vi "Monitor voltages.vi"() -> ()   [LabVIEW 2020]
uses:
  <vilib>/Utility/error.llb/DialogType.ctl
  <vilib>/DAQmx/read.llb/DAQmx Read (Analog 1D Wfm NChan NSamp).vi
  <vilib>/DAQmx/create/channels.llb/DAQmx Create Channel (AI-Voltage-Basic).vi
  <vilib>/DAQmx/configure/timing.llb/DAQmx Timing (Sample Clock).vi
  <vilib>/DAQmx/miscellaneous.llb/DAQmx Fill In Error Info.vi
  <vilib>/Utility/file.llb/Write Delimited Spreadsheet (DBL).vi
  <resource>/objmgr/daqmx.rc
  <vilib>/Analysis/NI_AALBase.lvlib
panel:
  out "Waveform Chart":cluster{"[0]":dbl, "[1]":dbl, "[2]":dbl}(graph)
  out "STD":dbl[](array[numeric])=[0.0007136534746484955, 0.0006582648996476653, 0.0006977354612249226]
  out "Mean voltage":dbl[](array[numeric])=[-1.226623991867514, -1.2306075649591512, -1.3978613305300918]
  in  "Log data":bool
  in  "Logging period (s)":dbl=1.0 caption="Time Target (s)"
  out "Waveform Graph":waveform(dbl)[](graph)=[{"t0"=timestamp(3798561010.450787 s since 1904-01-01), "dt"=0.001, "Y"=[-1.2267769584961297, -1.2264549234868314, -1.2259718709735348, -1.2267769584961297, -1.2254888184610193, -1.227904081031412, -1.2256498359651042, -1.2254888184610193, -1.2270989935057757, -1.227904081031412, -1.2264549234868314, -1.226615940991437, -1.226615940991437, -1.2275820460208966, -1.226615940991437, -1.2250057659492843, -1.2280650985368, -1.226615940991437, -1.2258108534692762, -1.2269379760009091, -1.2274210285157692, -1.2269379760009091, -1.2261328884778802, -1.2264549234868314, -1.2270989935057757, -1.2264549234868314, -1.2274210285157692, -1.2261328884778802, -1.2269379760009091, -1.2261328884778802, -1.2264549234868314, -1.2280650985368, -1.2264549234868314, -1.2267769584961297, -1.2270989935057757, -1.2269379760009091, -1.2267769584961297, -1.2270989935057757, -1.2259718709735348, -1.2269379760009091, -1.227260011010729, -1.2259718709735348, -1.2262939059823121, -1.2270989935057757, -1.2269379760009091, -1.226615940991437, -1.2259718709735348, -1.226615940991437, -1.2267769584961297, -1.2264549234868314, -1.2250057659492843, -1.2254888184610193, -1.2270989935057757, -1.2262939059823121, -1.225327800957021, -1.2277430635261108, -1.227260011010729, -1.2258108534692762, -1.2254888184610193, -1.2261328884778802, -1.2262939059823121, -1.2270989935057757, -1.2261328884778802, -1.227260011010729, -1.2254888184610193, -1.2258108534692762, -1.2277430635261108, -1.2280650985368, -1.2270989935057757, -1.2262939059823121, -1.2264549234868314, -1.226615940991437, -1.2264549234868314, -1.2269379760009091, -1.2269379760009091, -1.227904081031412, -1.2275820460208966, -1.2264549234868314, -1.2267769584961297, -1.2270989935057757, -1.2267769584961297, -1.2259718709735348, -1.2264549234868314, -1.2277430635261108, -1.2251667834531093, -1.2254888184610193, -1.2264549234868314, -1.2267769584961297, -1.2270989935057757, -1.2250057659492843, -1.2274210285157692, -1.226615940991437, -1.2264549234868314, -1.226615940991437, -1.2262939059823121, -1.2269379760009091, -1.226615940991437, -1.226615940991437, -1.2274210285157692, -1.2267769584961297], "attributes"=variant("NI_ChannelName"=variant(string "Dev1/ai0"), "NI_UnitDescription"=variant(string "Volts"))}, {"t0"=timestamp(3798561010.450798 s since 1904-01-01), "dt"=0.001, "Y"=[-1.2311244311557337, -1.2311244311557337, -1.230802396141731, -1.2299973086082525, -1.2312854486628662, -1.230802396141731, -1.2312854486628662, -1.2316074836773934, -1.230319343621382, -1.2306413786348607, -1.230802396141731, -1.2309634136486887, -1.2301583261147735, -1.2304803611280777, -1.2314464661700861, -1.230802396141731, -1.229675273595472, -1.2312854486628662, -1.230802396141731, -1.2298362911018186, -1.2304803611280777, -1.2306413786348607, -1.2301583261147735, -1.230319343621382, -1.2309634136486887, -1.230319343621382, -1.2298362911018186, -1.2306413786348607, -1.2309634136486887, -1.2295142560892127, -1.2298362911018186, -1.2309634136486887, -1.2306413786348607, -1.2301583261147735, -1.231768501184788, -1.230319343621382, -1.2306413786348607, -1.2299973086082525, -1.2298362911018186, -1.230319343621382, -1.2295142560892127, -1.2319295186922703, -1.2316074836773934, -1.2309634136486887, -1.2304803611280777, -1.2312854486628662, -1.230802396141731, -1.2293532385830404, -1.2304803611280777, -1.2322515537074974, -1.2306413786348607, -1.230802396141731, -1.2309634136486887, -1.2311244311557337, -1.2306413786348607, -1.2295142560892127, -1.2304803611280777, -1.2309634136486887, -1.2299973086082525, -1.2304803611280777, -1.2304803611280777, -1.230802396141731, -1.230802396141731, -1.2309634136486887, -1.2309634136486887, -1.2298362911018186, -1.2301583261147735, -1.2306413786348607, -1.2299973086082525, -1.230319343621382, -1.230802396141731, -1.2309634136486887, -1.2299973086082525, -1.2301583261147735, -1.228870186065047, -1.231768501184788, -1.2306413786348607, -1.230319343621382, -1.2304803611280777, -1.2290312035709576, -1.2306413786348607, -1.2312854486628662, -1.2295142560892127, -1.2309634136486887, -1.2316074836773934, -1.230802396141731, -1.2298362911018186, -1.230319343621382, -1.23209053619984, -1.2312854486628662, -1.2295142560892127, -1.2306413786348607, -1.231768501184788, -1.230802396141731, -1.230802396141731, -1.2306413786348607, -1.2299973086082525, -1.2298362911018186, -1.2312854486628662, -1.2312854486628662], "attributes"=variant("NI_ChannelName"=variant(string "Dev1/ai1"), "NI_UnitDescription"=variant(string "Volts"))}, {"t0"=timestamp(3798561010.450809 s since 1904-01-01), "dt"=0.001, "Y"=[-1.3980996365889728, -1.398743707022256, -1.3976165837651384, -1.3974555661574082, -1.3982606541971323, -1.3977776013729755, -1.3997098126754064, -1.3982606541971323, -1.3977776013729755, -1.3979386189809204, -1.3980996365889728, -1.3980996365889728, -1.398582689413774, -1.3977776013729755, -1.3980996365889728, -1.3997098126754064, -1.3980996365889728, -1.3971335309422703, -1.3980996365889728, -1.3980996365889728, -1.3979386189809204, -1.396972513334862, -1.396972513334862, -1.3990657422395425, -1.3984216718053992, -1.395845390086009, -1.3963284429063025, -1.398582689413774, -1.3968114957275615, -1.3976165837651384, -1.3980996365889728, -1.396972513334862, -1.3976165837651384, -1.3979386189809204, -1.396972513334862, -1.3979386189809204, -1.3980996365889728, -1.3977776013729755, -1.3980996365889728, -1.3971335309422703, -1.398743707022256, -1.3980996365889728, -1.3982606541971323, -1.3977776013729755, -1.3982606541971323, -1.3972945485497856, -1.3977776013729755, -1.3980996365889728, -1.3974555661574082, -1.3972945485497856, -1.3990657422395425, -1.398582689413774, -1.3971335309422703, -1.3982606541971323, -1.3997098126754064, -1.3972945485497856, -1.396650478120368, -1.3977776013729755, -1.398743707022256, -1.3984216718053992, -1.3979386189809204, -1.3979386189809204, -1.3982606541971323, -1.3979386189809204, -1.398582689413774, -1.3989047246308455, -1.3971335309422703, -1.396972513334862, -1.3974555661574082, -1.3972945485497856, -1.3979386189809204, -1.398582689413774, -1.3976165837651384, -1.3972945485497856, -1.3971335309422703, -1.3979386189809204, -1.3974555661574082, -1.396972513334862, -1.3984216718053992, -1.3976165837651384, -1.3964894605132818, -1.3982606541971323, -1.398582689413774, -1.3977776013729755, -1.3971335309422703, -1.3974555661574082, -1.3974555661574082, -1.3976165837651384, -1.3977776013729755, -1.3989047246308455, -1.3976165837651384, -1.396972513334862, -1.3982606541971323, -1.3984216718053992, -1.3979386189809204, -1.3972945485497856, -1.3976165837651384, -1.3972945485497856, -1.3977776013729755, -1.398743707022256], "attributes"=variant("NI_ChannelName"=variant(string "Dev1/ai2"), "NI_UnitDescription"=variant(string "Volts"))}]
  in  "Stop":bool
  in  "Number of Samples":i32=100
  in  "Save File Path":path=path "G:/Shared drives/PHYS - Walsworth Group/Experiment folders/Dark Matter/Confocal/Data/Nanostage monitoring/test.lvm"
  in  "Sample Rate":dbl=1000.0
  in  "Sample Clock Source":tag="OnboardClock"
  in  "Terminal Configuration":i32(ring)=-1 items=["default"=-1, "RSE"=10083, "NRSE"=10078, "Differential"=10106, "Pseudodifferential"=12529]
  in  "Max Voltage":dbl=10.0
  in  "Min Voltage":dbl=-10.0
  in  "Physical Channel":tag="Dev1/ai0:2"
  out "Actual Sample Rate":dbl=1000.0 format="%0.2f"
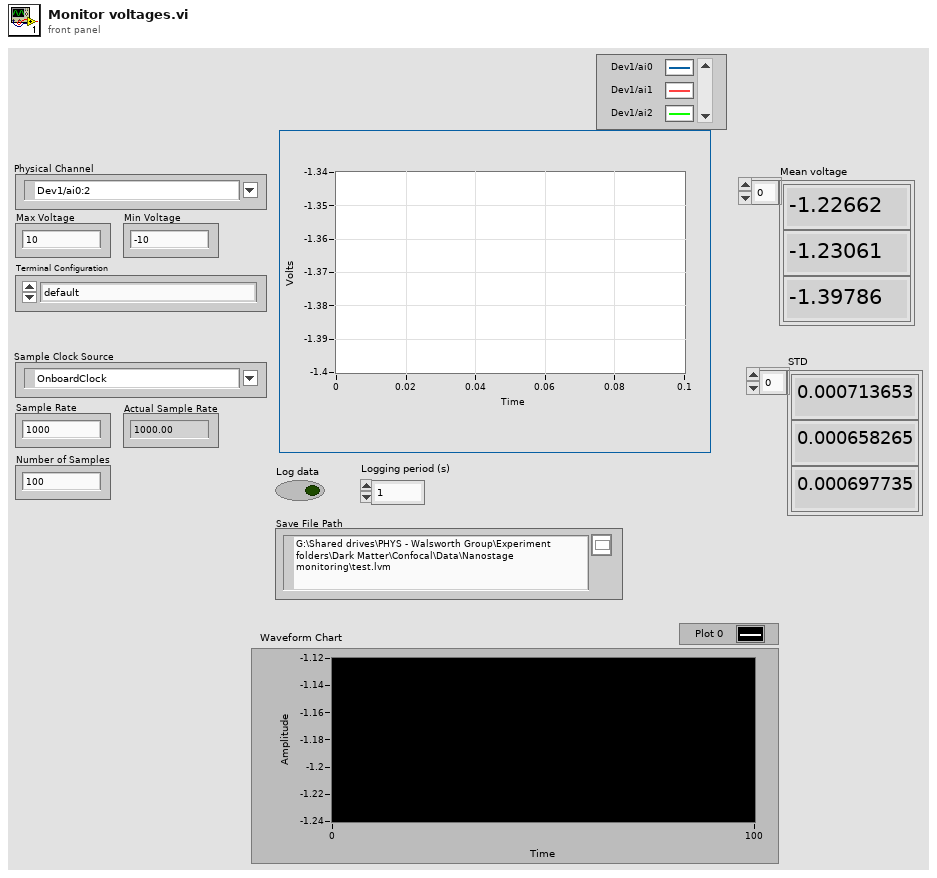
[diagram p1: front panel]
types:
  T1 = typedef "DialogType.ctl" = u16
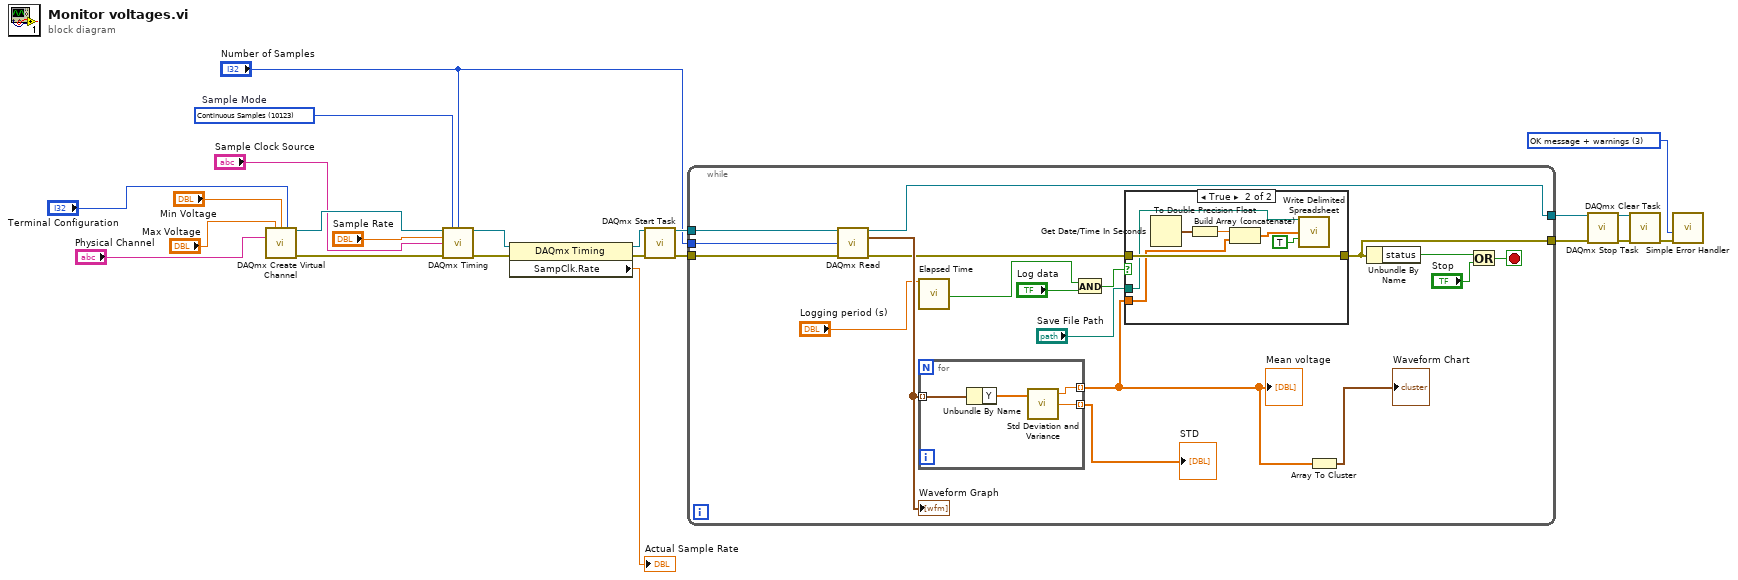
[diagram p0: block diagram]
diagram:
  w2 = T1 3 items=["no dialog", "OK message", "continue or stop message", "OK message + warnings", "continue/stop + warnings"] ("type of dialog (OK msg:1)")
  w21 = 10123 items=["Finite Samples"=10178, "Continuous Samples"=10123, "Hardware Timed Single Point"=12522]  # Sample Mode
  n1 = call-poly <vilib>:"DAQmx Create Virtual Channel.vi"("maximum value"="Max Voltage", "minimum value"="Min Voltage", "input terminal configuration"="Terminal Configuration", "physical channels"="Physical Channel") -> ("task out"=w19:refnum<k21>, "error out"=w20:errorcluster)  [unwired: 10 in]
  n2 = call-poly <vilib>:"DAQmx Timing.vi"("task/channels in"=w19, "sample mode"=w21, "samples per channel"="Number of Samples", "rate"="Sample Rate", "source"="Sample Clock Source", "error in"=w20) -> ("task out"=w23:refnum<k21>, "error out"=w22:errorcluster)  [unwired: 8 in]
  n3 = property class="DAQmx Timing"(reference=w23, error in=w22) -> (reference out=w1:refnum<k21>, error out=w18:errorcluster, "SampClk.Rate"=→"Actual Sample Rate":dbl)
  n4 = call <vilib>:"DAQmx Start Task.vi"("task/channels in"=w1, "error in"=w18) -> ("task out"=w17:refnum<k21>, "error out"=w16:errorcluster)  [unwired: 12 in]
  n5 = while {
    tunnel: w17 -> [w41]
    tunnel: w16 -> [w40]
    tunnel: [w39] -> w6
    tunnel: [w31] -> w5
    tunnel: "Number of Samples" -> [w35]
    stop <- w36 stop-if-true
    n6 = call-poly <vilib>:"DAQmx Read.vi"("task/channels in"=w41, "number of samples per channel"=w35, "error in"=w40) -> ("task out"=w39:refnum<k21>, "data"=w33:waveform(dbl)[], "error out"=w32:errorcluster)  [unwired: 10 in]
    "Waveform Graph" <- w33
    n7 = call "Elapsed Time"("Time Target (s)"="Logging period (s)") -> ("Time has Elapsed"=w29:bool)  [unwired: 11 in, 7 out]
    n8 = for {
      tunnel: w33 -> [w45] mode=indexing
      tunnel: [w43] -> w25 mode=indexing
      tunnel: [w42] -> w26 mode=indexing
      n9 = Unbundle By Name(w45) -> ("Y"=w44:dbl[])
      n10 = call <vilib>:"Std Deviation and Variance.vi"("X"=w44) -> ("mean"=w43:dbl, "standard deviation"=w42:dbl)  [unwired: 1 in, 1 out]
    }
    "Mean voltage" <- w25
    "STD" <- w26
    n11 = And(x=w29, y="Log data") -> (x .and. y?=w27:bool)
    n12 = case shown="True" w27 {
      tunnel: "Save File Path" -> [_ w49]
      tunnel: w32 -> [w46 w53]
      tunnel: [w46 w53] -> w31
      tunnel: w25 -> [_ w47]
      frame False {
      }
      frame True {
        n13 = Get Date/Time In Seconds() -> (seconds since 1Jan1904=w52:timestamp)
        n14 = To Double Precision Float(number=w52) -> (double precision float=w51:dbl)
        n15 = Build Array (concatenate)(w51, w47) -> (w50:dbl[])
        n16 = call-poly <vilib>:"Write Delimited Spreadsheet.vi"("file path (dialog if empty)"=w49, "1D data"=w50, "append to file? (new file:F)"=TRUE) -> ()  [unwired: 11 in, 2 out]
      }
    }
    n17 = Array To Cluster(array=w25) -> (cluster=→"Waveform Chart":cluster{"[0]":dbl, "[1]":dbl, "[2]":dbl})
    n18 = Unbundle By Name(w31) -> ("status"=w37:bool)
    n19 = Or(x=w37, y="Stop") -> (x .or. y?=w36:bool)
  }
  n20 = call <vilib>:"DAQmx Stop Task.vi"("task/channels in"=w6, "error in"=w5) -> ("task out"=w3:refnum<k21>, "error out"=w4:errorcluster)  [unwired: 12 in]
  n21 = call <vilib>:"DAQmx Clear Task.vi"("task in"=w3, "error in"=w4) -> ("error out"=w15:errorcluster)  [unwired: 13 in]
  n22 = call <vilib>:"Simple Error Handler.vi"("type of dialog (OK msg:1)"=w2, "error in (no error)"=w15) -> ()  [unwired: 3 in, 5 out]
